vi "iV programa 2_3.vi"() -> ()   [LabVIEW 2020]
panel:
  out "time 2":i32
  out "Thermometer":dbl(slide) scale=0.0..100.0
  out "time Seconds":i32
  out "Tank":dbl(slide) scale=0.0..10.0
  # "2.3. Simulación de un proceso. Considere lo siguiente:\n• Elabore un programa que simule el llenado de un tanque en un tiempo de 10 segundos. (Queda a su consideración los incrementos)\n• Una vez que ha sido llenado el tanque. Simule el aumento de la temperatura de 25 grados a 90 grados en un tiempo aproximado de 15 segundos. (Queda a su consideración los incrementos).\n• Al llegar a la temperatura de 90 grados, deberá mostrar una alerta visual y habilitar una opción que permita finalizar el proceso por el usuario."
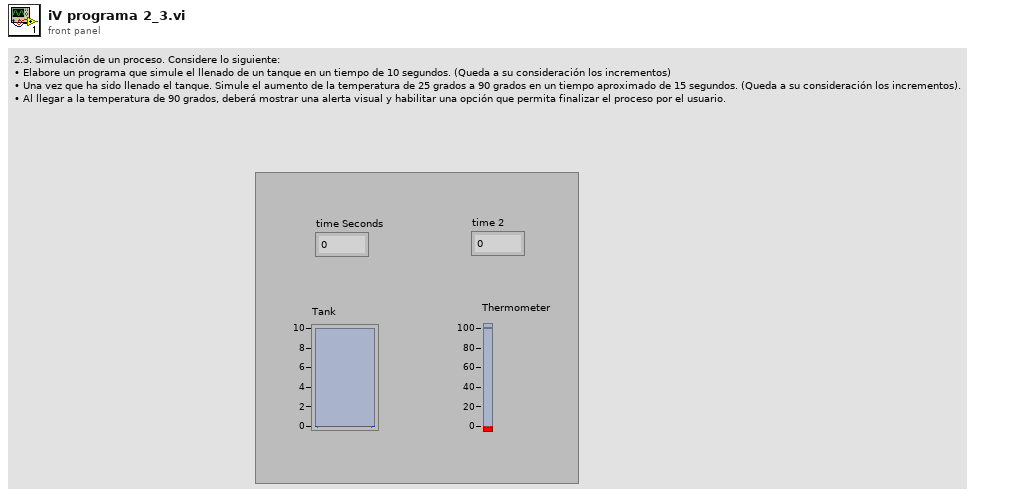
[diagram p1: front panel]
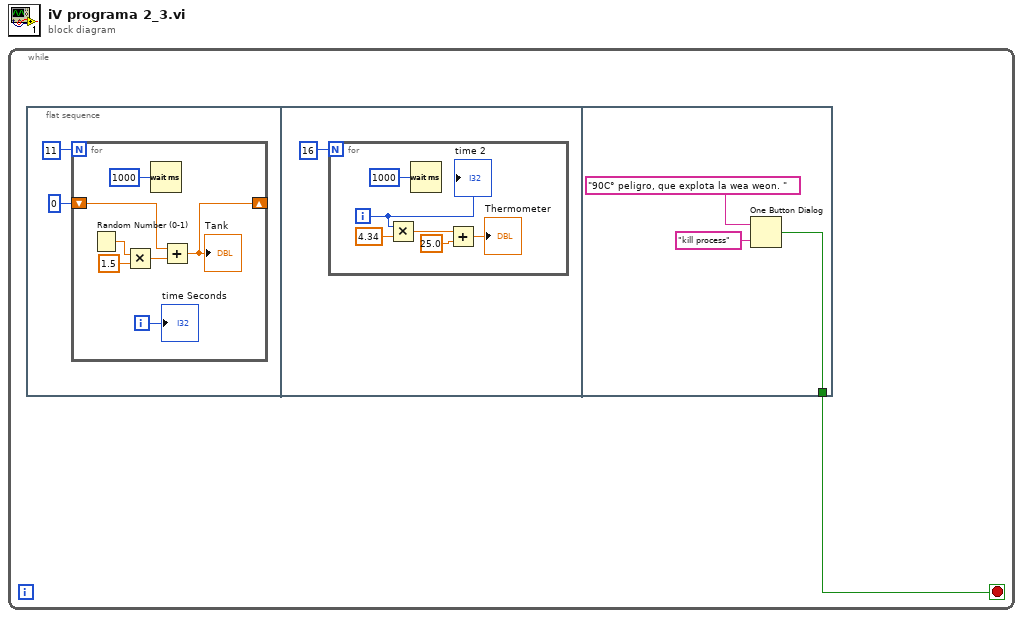
[diagram p0: block diagram]
diagram:
  n1 = while {
    stop <- w1 stop-if-true
    n2 = flat-sequence {
      tunnel: [w18] -> w1
      frame #0 {
        n3 = for {
          N: 11 -> [_]
          shift-right: [w8] -> _
          shift-left: 0 -> [w9]
          i -> [w10]
          n4 = Random Number (0-1)() -> (number: 0 to 1=w7:dbl)
          n5 = Multiply(x=w7, y=1.5) -> (x*y=w5:dbl)
          n6 = Wait (ms)(milliseconds to wait=u32 1000) -> ()  [unwired: 1 out]
          n7 = Add(x=w9, y=w5) -> (x+y=w8:dbl)
          "Tank" <- w8
          "time Seconds" <- w10
        }
      }
      frame #1 {
        n8 = for {
          N: 16 -> [_]
          i -> [w17]
          n9 = Multiply(x=w17, y=4.34) -> (x*y=w15:dbl)
          n10 = Wait (ms)(milliseconds to wait=u32 1000) -> ()  [unwired: 1 out]
          n11 = Add(x=w15, y=25.0) -> (x+y=→"Thermometer":dbl)
          "time 2" <- w17
        }
      }
      frame #2 {
        n12 = One Button Dialog(message="90C° peligro, que explota la wea weon. ", button name ("OK")="kill process") -> (true=w18:bool)
      }
    }
  }
